vi "KeywordWriteIfDifferent.vi"(0 "Crate":string, 2 "Keyword":string, 3 "Value":string, 7 "Service":string, 9 "error in (no error)":errorcluster) -> (1 "done?":refnum<k4>, 6 "error out":errorcluster)   [LabVIEW 2009]
uses:
  Controls/KeywordCommand.ctl
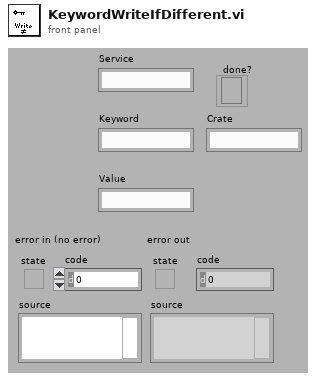
[diagram p1: front panel]
types:
  T1 = typedef "KeywordCommand.ctl" = cluster{"Command":enum16{"READ", "READBINARY", "WRITE", "QUIT"}, "Service":string, "Keyword":string, "Value":string, "done?":refnum<k4>}
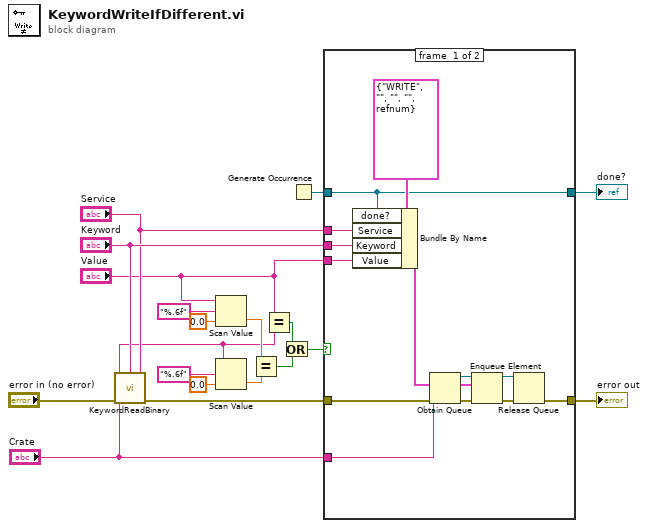
[diagram p0: block diagram]
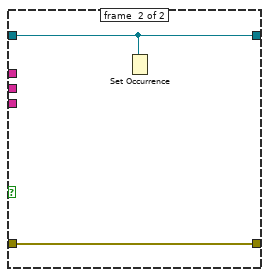
[diagram p2: hidden frame]
diagram:
  n1 = call "KeywordReadBinary.vi"("Service"="Service", "Keyword"="Keyword", "Crate"="Crate", "error in (no error)"="error in (no error)") -> ("Value"=w1:string, "error out"=w18:errorcluster)  [unwired: 4 out]
  n2 = Scan Value(string="Value", format string="%.6f", default (0 dbl)=0.0 ("default (0 I32)")) -> (value=w9:dbl)  [unwired: 1 out]
  n3 = Scan Value(string=w1, format string="%.6f", default (0 dbl)=0.0 ("default (0 I32)")) -> (value=w2:dbl)  [unwired: 1 out]
  n4 = Equal?(x=w9, y=w2) -> (x = y?=w8:bool)
  n5 = Equal?(x="Value", y=w1) -> (x = y?=w7:bool)
  n6 = Or(x=w7, y=w8) -> (x .or. y?=w6:bool)
  n7 = Generate Occurrence() -> (w14:refnum<k4>)
  n8 = case shown="False" w6 {
    tunnel: w18 -> [w26 w34]
    tunnel: "Crate" -> [w25 _]
    tunnel: "Keyword" -> [w24 _]
    tunnel: "Service" -> [w23 _]
    tunnel: "Value" -> [w22 _]
    tunnel: w14 -> [w21 w33]
    tunnel: [w21 w33] -> w13
    tunnel: [w20 w34] -> w12
    frame #0 {
      n9 = Bundle By Name(cluster=T1 {"Command"=enum."WRITE", "Service"="", "Keyword"="", "Value"="", "done?"=refnum} ("KeywordCommand"), "done?"=w21, "Service"=w23, "Keyword"=w24, "Value"=w22) -> (w29:T1)
      n10 = Obtain Queue(name (unnamed)=w25, element data type=w29, error in (no error)=w26) -> (queue out=w30:refnum<queue>, error out=w31:errorcluster)  [unwired: 2 in, 1 out]
      n11 = Enqueue Element(queue=w30, element=w29, error in (no error)=w31) -> (queue out=w27:refnum<queue>, error out=w28:errorcluster)  [unwired: 2 out]
      n12 = Release Queue(queue=w27, error in (no error)=w28) -> (error out=w20:errorcluster)  [unwired: 3 out]
    }
    frame #1 {
      n13 = Set Occurrence(w33) -> ()
    }
  }
  "done?" <- w13
  "error out" <- w12
